vi "Frame Code Status Display.vi"(0 "Status":bool, 5 "Complete":bool, 7 "SN":string, 9 "Frame":string, 11 "error in (no error)":errorcluster) -> (4 "information":T1, 15 "error out":errorcluster)   [LabVIEW 2014]
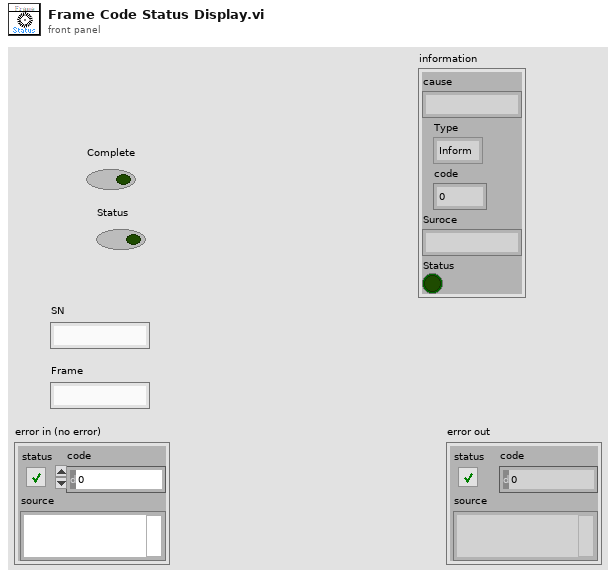
[diagram p1: front panel]
types:
  T1 = cluster{"cause":string, "Type":enum16{"Inform", "Warning", "Alarm"}, "code":i32, "Suroce":string, "Status":bool}
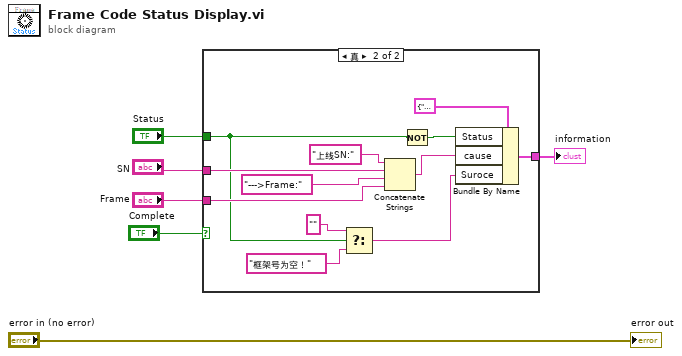
[diagram p0: block diagram]
diagram:
  n1 = case shown="真" "Complete" {
    tunnel: "Status" -> [_ w10]
    tunnel: "SN" -> [_ w16]
    tunnel: "Frame" -> [_ w15]
    tunnel: [_ w13] -> w2
    frame False {
    }
    frame True {
      n2 = Select(t="", s=w10, f="框架号为空！") -> (s? t:f=w8:string)
      n3 = Concatenate Strings("上线SN:", w16, "--->Frame:", w15) -> (w14:string)
      n4 = Not(x=w10) -> (.not. x?=w11:bool)
      n5 = Bundle By Name(cluster=T1 {"cause"="", "Type"=enum."Inform", "code"=0, "Suroce"="", "Status"=FALSE} ("information"), "Status"=w11, "cause"=w14, "Suroce"=w8) -> (w13:T1)
    }
  }
  "information" <- w2
  "error out" <- "error in (no error)"
